vi "RTEH Init.vi"(8 "error in (no error)":errorcluster, 10 "Number of Priorities":i32=3, 11 "Notifications per Priority":i32=5) -> (0 "error out":errorcluster)   [LabVIEW 2017]
doc: "This VI initializes the notification queue used to transfer errors from Specific Error Handler instances to the Central Error Handler. \n\nThe notification queue is a priority queue where each priority has a fixed number of entries. Elements are always removed from the highest priority available. Priorities are specified in a lowest-to-highest order, so priority 0 is the highest priority and priority Number of Priorities-1 is the lowest.\n\nYou only need to call this VI if you are using error notification.\n\nThis VI is optimized for Real-Time applications. An alternate version for Windows VIs exists."
uses:
  <userlib>/_SEH/Controls/Shared/SEH Error Notification Command.ctl
  <userlib>/_SEH/Controls/Shared/SEH Error Notification Config.ctl
  <userlib>/_SEH/Controls/RTEH/RTEH Status Type.ctl
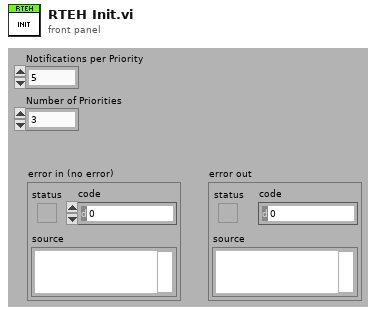
[diagram p1: front panel]
types:
  T1 = typedef "SEH Error Notification Config.ctl" = cluster{"Number of Priorities":i32, "Notifications per Priority":i32}
  T2 = typedef "SEH Error Notification Command.ctl" = enum16{"Init", "Send Error", "Check Error", "Invalid Command"}
  T3 = typedef "RTEH Status Type.ctl" = enum16{"Success", "Error", "Warning", "Skipped Notification"}
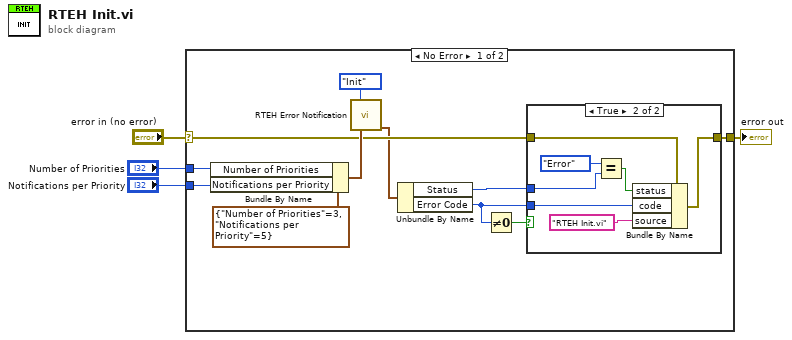
[diagram p0: block diagram]
diagram:
  n1 = case shown="No Error" "error in (no error)" {
    selector: "error in (no error)" -> [w10 w24]
    tunnel: "Number of Priorities" -> [w12 _]
    tunnel: "Notifications per Priority" -> [w11 _]
    tunnel: [w9 w24] -> w1
    frame No Error {
      n2 = Bundle By Name(cluster=T1 {"Number of Priorities"=3, "Notifications per Priority"=5} ("Configuration"), "Number of Priorities"=w12, "Notifications per Priority"=w11) -> (w13:T1)
      n3 = call <userlib>:"RTEH Error Notification.vi"("Command"=SEH_Error_Notification_Command."Init", "Configuration"=w13) -> ("Internal Status"=w8:cluster{"Status":T3, "Error Code":i32})  [unwired: 6 in, 7 out]
      n4 = Unbundle By Name(w8) -> ("Status"=w7:T3, "Error Code"=w6:i32)
      n5 = Not Equal To 0?(x=w6) -> (x != 0?=w5:bool)
      n6 = case shown="True" w5 {
        tunnel: w10 -> [w16 w23]
        tunnel: [w16 w22] -> w9
        tunnel: w6 -> [_ w21]
        tunnel: w7 -> [_ w20]
        frame False {
        }
        frame True {
          n7 = Equal?(x=RTEH_Status_Type."Error", y=w20) -> (x = y?=w19:bool)
          n8 = Bundle By Name(cluster=w23, "status"=w19, "code"=w21, "source"="RTEH Init.vi") -> (w22:errorcluster)
        }
      }
    }
    frame Error {
    }
  }
  "error out" <- w1
